vi "Host Main.vi"() -> ()   [LabVIEW 2014]
uses:
  <vilib>/robotics/Controls/2D Rangefinder/NI_Robotics_2D Rangefinder.xctl
  <vilib>/robotics/TaimiOmni/TaimiOmni/TaimiOmniIRDataArray.ctl
  <vilib>/robotics/TaimiOmni/TaimiOmni/TaimiOmniIRData.ctl
  <vilib>/Utility/inputDevices.llb/joystickAcquire.vi
  <vilib>/Utility/inputDevices.llb/closeJoystick.vi
  <vilib>/robotics/TaimiOmni/TaimiOmni/TaimiOmni.lvclass
panel:
  in  "device index":i32
  out "end":bool
  in  "IP Address":string="172.22.11.2"
  in  "Y Velocity (m/s)":dbl(slide) min=-1.0 max=1.0 scale=-0.3..0.3
  out "Y Velocity Feedback":dbl(slide) scale=-0.3..0.3
  in  "X Velocity (m/s)":dbl(slide) min=-1.0 max=1.0 scale=-0.3..0.3
  out "X Velocity Feedback":dbl(slide) scale=-0.3..0.3
  in  "Angular Velocity (rad/s)":dbl(slide) min=-2.0 max=2.0 scale=2.0..-2.0
  out "Angular Velocity Feedback":dbl(slide) scale=2.0..-2.0
  in  "stop":bool
  in  "Break":bool
  out "Robot Status:":string
  out "IR Distances":cluster{"angle":dbl[], "distance":dbl[][]}(xcontrol)
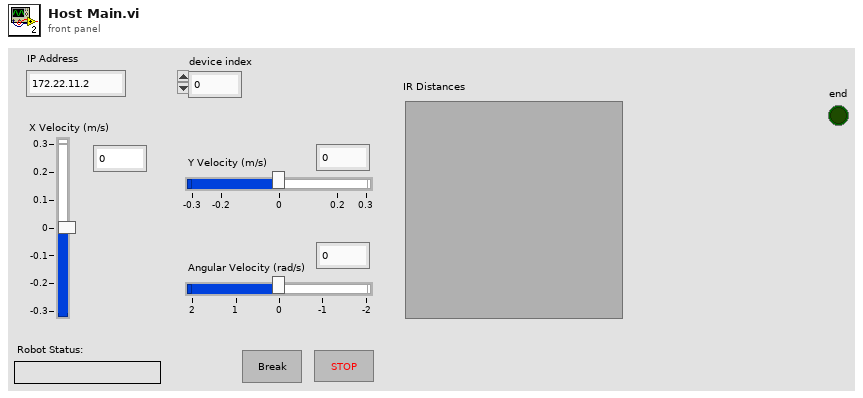
[diagram p1: front panel]
types:
  T1 = cluster{"Read Access":enum8{"Allowed", "Required", "None"}, "Write Access":enum8{"Allowed", "Required", "None"}}
  T2 = typedef "TaimiOmni.lvclass/TaimiOmniIRDataArray.ctl" = T3[]
  T3 = typedef "TaimiOmni.lvclass/TaimiOmniIRData.ctl" = cluster{"distance":dbl, "angle":dbl}
  T4 = cluster{"X axis":i32, "Y axis":i32, "Z axis":i32, "X axis rotation":i32, "Y axis rotation":i32, "Z axis rotation":i32, "U axis":i32, "V axis":i32}
  T5 = cluster{"button 1":bool, "button 2":bool, "button 3":bool, "button 4":bool, "button 5":bool, "button 6":bool, "button 7":bool, "button 8":bool, "button 9":bool, "button 10":bool, "button 11":bool, "button 12":bool, "button 13":bool, "button 14":bool, "button 15":bool, "button 16":bool, "button 17":bool, "button 18":bool, "button 19":bool, "button 20":bool, "button 21":bool, "button 22":bool, "button 23":bool, "button 24":bool, "button 25":bool, "button 26":bool, "button 27":bool, "button 28":bool, "button 29":bool, "button 30":bool, "button 31":bool, "button 32":bool}
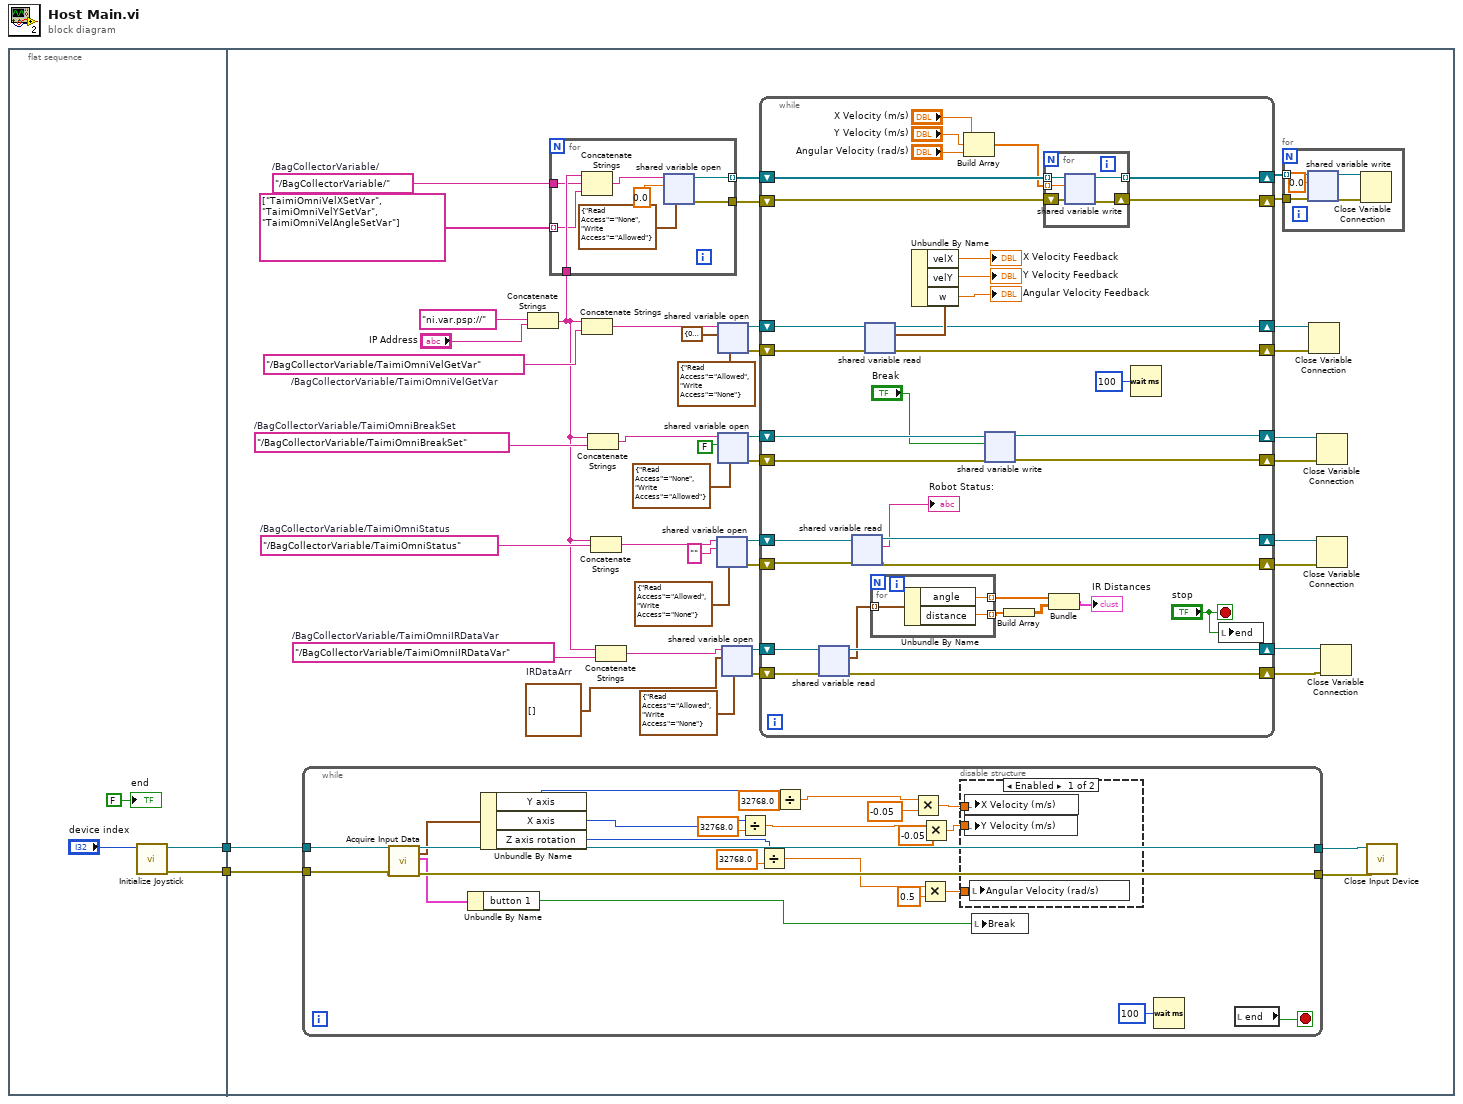
[diagram p0: block diagram]
diagram:
  n1 = flat-sequence {
    tunnel: [w5] -> w2
    tunnel: [w4] -> w1
    tunnel: w2 -> [w10]
    tunnel: w1 -> [w9]
    frame #0 {
      n2 = call <vilib>:"Initialize Joystick.vi"("device index"="device index") -> ("error out"=w4:errorcluster, "device ID"=w5:refnum<k1>)  [unwired: 9 in]
      "end" <- FALSE ("end")
    }
    frame #1 {
      w15 = T2 []  # IRDataArr
      w16 = "/BagCollectorVariable/TaimiOmniIRDataVar"  # /BagCollectorVariable/TaimiOmniIRDataVar
      w25 = "/BagCollectorVariable/TaimiOmniStatus"  # /BagCollectorVariable/TaimiOmniStatus
      w34 = "/BagCollectorVariable/TaimiOmniBreakSet"  # /BagCollectorVariable/TaimiOmniBreakSet
      w45 = "/BagCollectorVariable/"  # /BagCollectorVariable/
      w47 = "/BagCollectorVariable/TaimiOmniVelGetVar"  # /BagCollectorVariable/TaimiOmniVelGetVar
      n3 = while {
        tunnel: w10 -> [w73]
        tunnel: w9 -> [w72]
        tunnel: [w71] -> w8
        tunnel: [w70] -> w7
        stop <- w75 stop-if-true
        n4 = call-poly <vilib>:"Acquire Input Data.vi"("device ID"=w73, "error in (no error)"=w72) -> ("device ID"=w71:refnum<k1>, "axis info"=w69:T4, "button info"=w62:T5, "error out"=w70:errorcluster)  [unwired: 13 in, 1 out]
        n5 = Unbundle By Name(w62) -> ("button 1"=w61:bool)
        n6 = Unbundle By Name(w69) -> ("Y axis"=w59:i32, "X axis"=w56:i32, "Z axis rotation"=w53:i32)
        n7 = Divide(x=w56, y=32768.0) -> (x/y=w55:dbl)
        n8 = Divide(x=w53, y=32768.0) -> (x/y=w52:dbl)
        n9 = Divide(x=w59, y=32768.0) -> (x/y=w58:dbl)
        n10 = Multiply(x=w58, y=-0.05) -> (x*y=w67:dbl)
        n11 = Multiply(x=w52, y=0.5) -> (x*y=w63:dbl)
        n12 = Multiply(x=w55, y=-0.05) -> (x*y=w66:dbl)
        n13 = disable-structure shown="Enabled" {
          disable-tunnel: w67 -> [w78 _]
          disable-tunnel: w66 -> [w77 _]
          disable-tunnel: w63 -> [w76 _]
          frame Enabled {
            n14 = local write "X Velocity (m/s)"(w78) -> ()
            n15 = local write "Y Velocity (m/s)"(w77) -> ()
            n16 = local write "Angular Velocity (rad/s)"(w76) -> ()
          }
          frame Disabled {
          }
        }
        n17 = local write "Break"(w61) -> ()
        n18 = Wait (ms)(milliseconds to wait=u32 100) -> ()  [unwired: 1 out]
        n19 = local read "end"() -> (w75:bool)
      }
      n20 = Concatenate Strings("ni.var.psp://" ("string"), "IP Address") -> (w17:string)
      n21 = for {
        tunnel: w17 -> [w91]
        tunnel: w45 -> [w90]
        tunnel: [w87] -> w44 mode=indexing
        tunnel: [w86] -> w41
        tunnel: string[] ["TaimiOmniVelXSetVar", "TaimiOmniVelYSetVar", "TaimiOmniVelAngleSetVar"] -> [w85] mode=indexing
        n22 = Concatenate Strings(w91, w90, w85) -> (w89:string)
        n23 = shared-variable-open(w89, 0.0 ("X Velocity (m/s)"), T1 {"Read Access"=enum."None", "Write Access"=enum."Allowed"} ("access")) -> (w87:refnum<k21>, w86:errorcluster)  [unwired: 1 in]
      }
      n24 = Concatenate Strings(w17, w47) -> (w46:string)
      n25 = Concatenate Strings(w17, w34) -> (w33:string)
      n26 = Concatenate Strings(w17, w25) -> (w27:string)
      n27 = Concatenate Strings(w17, w16) -> (w19:string)
      n28 = shared-variable-open(w27, "", T1 {"Read Access"=enum."Allowed", "Write Access"=enum."None"} ("access")) -> (w24:refnum<k21>, w23:errorcluster)  [unwired: 1 in]
      n29 = shared-variable-open(w46, cluster{"velX":dbl, "velY":dbl, "w":dbl} {"velX"=0.0, "velY"=0.0, "w"=0.0} ("input cluster"), T1 {"Read Access"=enum."Allowed", "Write Access"=enum."None"} ("access")) -> (w43:refnum<k21>, w42:errorcluster)  [unwired: 1 in]
      n30 = shared-variable-open(w33, FALSE, T1 {"Read Access"=enum."None", "Write Access"=enum."Allowed"} ("access")) -> (w32:refnum<k21>, w31:errorcluster)  [unwired: 1 in]
      n31 = shared-variable-open(w19, w15, T1 {"Read Access"=enum."Allowed", "Write Access"=enum."None"} ("access")) -> (w14:refnum<k21>, w13:errorcluster)  [unwired: 1 in]
      n32 = while {
        shift-right: [w120] -> w38
        shift-left: w44 -> [w122]
        shift-right: [w119] -> w37
        shift-left: w41 -> [w121]
        shift-right: [w114] -> w39
        shift-left: w42 -> [w117]
        shift-right: [w115] -> w40
        shift-left: w43 -> [w118]
        shift-right: [w108] -> w29
        shift-left: w32 -> [w111]
        shift-right: [w107] -> w28
        shift-left: w31 -> [w110]
        shift-right: [w104] -> w21
        shift-left: w24 -> [w106]
        shift-right: [w103] -> w20
        shift-left: w23 -> [w105]
        shift-right: [w99] -> w12
        shift-left: w14 -> [w101]
        shift-right: [w98] -> w11
        shift-left: w13 -> [w100]
        stop <- "stop" stop-if-true
        n33 = shared-variable-read(w101, w100) -> (w99:refnum<k21>, w98:errorcluster, w97:T2)  [unwired: 1 out]
        n34 = shared-variable-read(w106, w105) -> (w104:refnum<k21>, w103:errorcluster, →"Robot Status:":string)  [unwired: 1 out]
        n35 = shared-variable-read(w118, w117) -> (w115:refnum<k21>, w114:errorcluster, w116:cluster{"velX":dbl, "velY":dbl, "w":dbl})  [unwired: 1 out]
        n36 = for {
          tunnel: w97 -> [w131] mode=indexing
          tunnel: [w130] -> w96 mode=indexing
          tunnel: [w129] -> w95 mode=indexing
          n37 = Unbundle By Name(w131) -> ("angle"=w130:dbl, "distance"=w129:dbl)
        }
        n38 = Unbundle By Name(w116) -> ("velX"=→"X Velocity Feedback":dbl, "velY"=→"Y Velocity Feedback":dbl, "w"=→"Angular Velocity Feedback":dbl)
        n39 = Build Array("X Velocity (m/s)", "Y Velocity (m/s)", "Angular Velocity (rad/s)") -> (w112:dbl[])
        n40 = shared-variable-write(w111, w110, "Break") -> (w108:refnum<k21>, w107:errorcluster)
        n41 = Build Array(w95) -> (w94:dbl[][])
        n42 = for {
          tunnel: w122 -> [w136] mode=indexing
          tunnel: w112 -> [w132] mode=indexing
          tunnel: [w134] -> w120 mode=indexing
          shift-right: [w133] -> w119
          shift-left: w121 -> [w135]
          n43 = shared-variable-write(w136, w135, w132) -> (w134:refnum<k21>, w133:errorcluster)
        }
        n44 = Bundle(w96, w94) -> (→"IR Distances":cluster{dbl[], dbl[][]})  [unwired: 1 in]
        n45 = Wait (ms)(milliseconds to wait=u32 100) -> ()  [unwired: 1 out]
        n46 = local write "end"("stop") -> ()
      }
      n47 = for {
        tunnel: w38 -> [w83] mode=indexing
        tunnel: w37 -> [w82]
        n48 = shared-variable-write(w83, w82, 0.0 ("data in")) -> (w81:refnum<k21>, w80:errorcluster)
        n49 = Close Variable Connection(8:w80, 11:w81) -> ()  [unwired: 1 out]
      }
      n50 = Close Variable Connection(8:w39, 11:w40) -> ()  [unwired: 1 out]
      n51 = Close Variable Connection(8:w28, 11:w29) -> ()  [unwired: 1 out]
      n52 = Close Variable Connection(8:w20, 11:w21) -> ()  [unwired: 1 out]
      n53 = Close Variable Connection(8:w11, 11:w12) -> ()  [unwired: 1 out]
      n54 = call-poly <vilib>:"Close Input Device.vi"("error in (no error)"=w7, "device ID"=w8) -> ()  [unwired: 8 in, 1 out]
    }
  }
